vi "FTW-Actor-Child-Get.vi"(0 "FTW-ActorInstance In":refnum<class "FTW-ActorInstance.lvclass">, 5 "Connector Name":string, 11 "error in":errorcluster) -> (4 "FTW-ActorInstance Out":refnum<class "FTW-ActorInstance.lvclass">, 6 "FTW Actor Connector":refnum<class "FTW-ActorConnector.lvclass">, 15 "error out":errorcluster)   [LabVIEW 2015, in "FTW-ActorInstance.lvclass"]
uses:
  FTW-ActorInstance.lvclass
  Connector/FTW-ActorConnector.lvclass
  FTW-ActorInstance.lvclass/FTW-ActorInstance.ctl
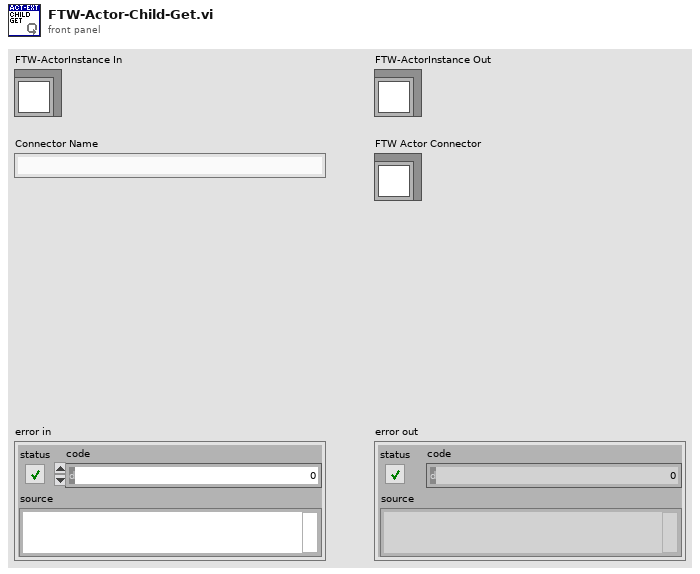
[diagram p1: front panel]
types:
  T1 = cluster{"Name":string, "URI":string, "Connector":refnum<class "FTW-ActorConnector.lvclass">, "Child":bool}[]
  T2 = cluster{"Name":string, "URI":string, "Connector":refnum<class "FTW-ActorConnector.lvclass">, "Child":bool}
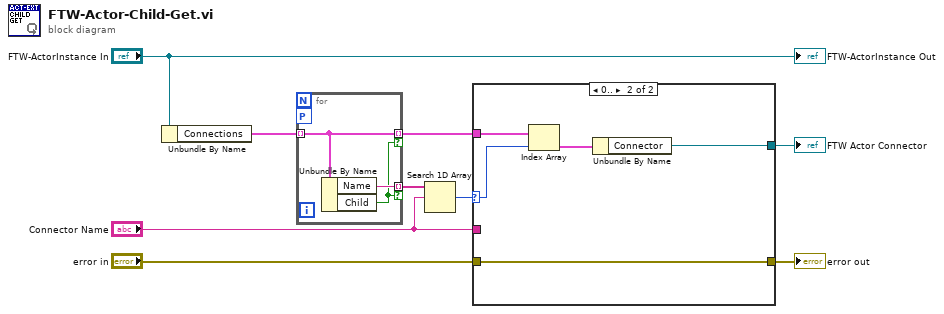
[diagram p0: block diagram]
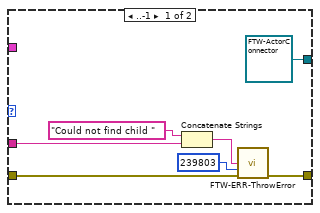
[diagram p2: hidden frame]
diagram:
  n1 = Unbundle By Name("FTW-ActorInstance In") -> ("Connections"=w7:T1)
  n2 = for {
    tunnel: w7 -> [w11] mode=indexing
    tunnel: [w12] -> w3 mode=indexing if=w10
    workers-P: _ -> [_]
    tunnel: [w11] -> w1 mode=indexing if=w10
    n3 = Unbundle By Name(w11) -> ("Name"=w12:string, "Child"=w10:bool)
  }
  n4 = Search 1D Array(1D array=w3, element="Connector Name") -> (index of element=w8:i32)  [unwired: 1 in]
  n5 = case shown="0.." w8 {
    selector: w8 -> [_ w24]
    tunnel: w1 -> [_ w23]
    tunnel: [w18 w22] -> w6
    tunnel: "error in" -> [w19 w22]
    tunnel: "Connector Name" -> [w14 _]
    tunnel: [refnum<class "FTW-ActorConnector.lvclass"> refnum ("Connector") w20] -> w2
    frame ..-1 {
      n6 = Concatenate Strings("Could not find child " ("Error Message"), w14) -> (w15:string)
      n7 = call "FTW-ERR-ThrowError.vi"("Error Message"=w15, "Error Code"=239803, "error in"=w19) -> ("error out"=w18:errorcluster)  [unwired: 12 in]
    }
    frame 0.. {
      n8 = Index Array(array=w23, index=w24) -> (element=w21:T2)
      n9 = Unbundle By Name(w21) -> ("Connector"=w20:refnum<class "FTW-ActorConnector.lvclass">)
    }
  }
  "error out" <- w6
  "FTW Actor Connector" <- w2
  "FTW-ActorInstance Out" <- "FTW-ActorInstance In"
